vi "Car-tracking-poc.vi"() -> ()   [LabVIEW 2026]
uses:
  CTI-Grove/Examples/Sourcecode/cti-drivers-lv-visa-simple/Examples/Driver/Public/Digital Direction.ctl
  CTI-Grove/Examples/Sourcecode/cti-drivers-lv-visa-simple/Examples/Driver/CTIPicoVISA.lvlib
panel:
  out "RIGHT":bool
  out "CENTRE":bool
  out "LEFT":bool
  out "Identity":T1
  in  "stop":bool
  in  "VISA resource name in":refnum<visa-resource-name>="ASRL1::INSTR"
  out "error out":errorcluster
  # "https://wiki.seeedstudio.com/Grove-Passive-Buzzer/"
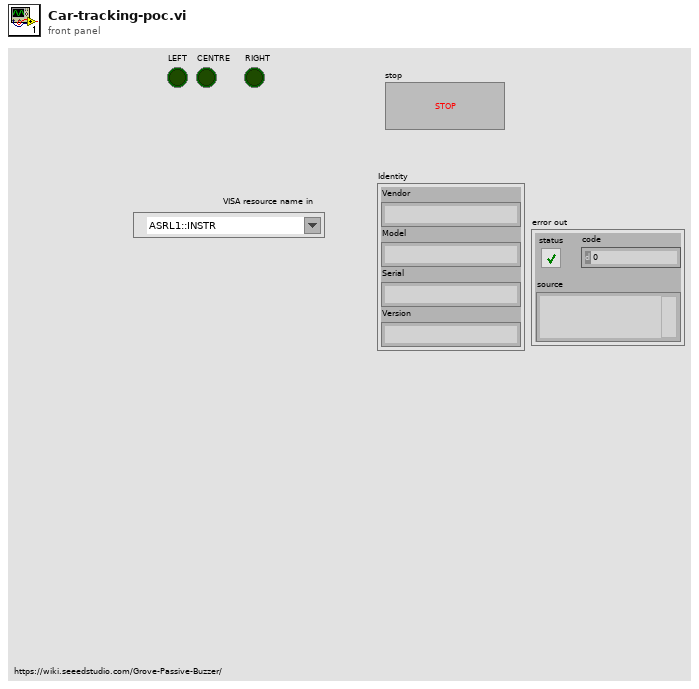
[diagram p1: front panel]
types:
  T1 = cluster{"Vendor":string, "Model":string, "Serial":string, "Version":string}
  T2 = typedef "CTIPicoVISA.lvlib/Digital Direction.ctl" = enum16{"In", "Out"}
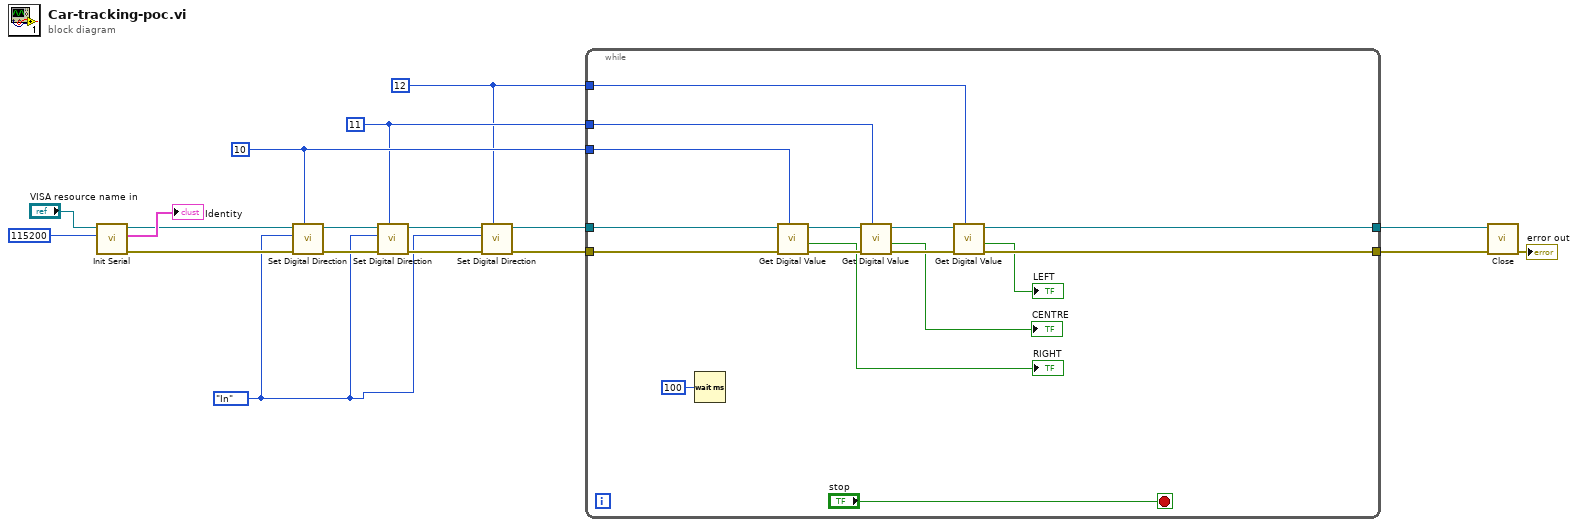
[diagram p0: block diagram]
diagram:
  w1 = 12 ("GPIO")
  w8 = 11 ("GPIO")
  w4 = Digital_Direction."In" ("Direction")
  w12 = 10 ("GPIO")
  n1 = call "Init Serial.vi"("Baud (115200)"=u32 115200, "VISA resource name in"="VISA resource name in") -> ("error out"=w13:errorcluster, "Identity"=→"Identity":T1, "VISA resource name Out"=w14:refnum<visa-resource-name>)  [unwired: 7 in]
  n2 = call "Set Digital Direction.vi"("GPIO"=w12, "error in (no error)"=w13, "Direction"=w4, "VISA resource name in"=w14) -> ("error out"=w10:errorcluster, "VISA resource name"=w11:refnum<visa-resource-name>)  [unwired: 6 in]
  n3 = call "Set Digital Direction.vi"("GPIO"=w8, "error in (no error)"=w10, "Direction"=w4, "VISA resource name in"=w11) -> ("error out"=w9:errorcluster, "VISA resource name"=w6:refnum<visa-resource-name>)  [unwired: 6 in]
  n4 = call "Set Digital Direction.vi"("GPIO"=w1, "error in (no error)"=w9, "Direction"=w4, "VISA resource name in"=w6) -> ("error out"=w7:errorcluster, "VISA resource name"=w5:refnum<visa-resource-name>)  [unwired: 6 in]
  n5 = while {
    tunnel: w12 -> [w22]
    tunnel: w5 -> [w32]
    tunnel: w7 -> [w28]
    tunnel: w8 -> [w23]
    tunnel: [w29] -> w3
    tunnel: [w25] -> w2
    tunnel: w1 -> [w24]
    stop <- "stop" stop-if-true
    n6 = Wait (ms)(milliseconds to wait=u32 100) -> ()  [unwired: 1 out]
    n7 = call "Get Digital Value.vi"("GPIO"=w22, "error in (no error)"=w28, "VISA resource name in"=w32) -> ("error out"=w27:errorcluster, "Value"=→"RIGHT":bool, "VISA resource name"=w31:refnum<visa-resource-name>)  [unwired: 6 in]
    n8 = call "Get Digital Value.vi"("GPIO"=w23, "error in (no error)"=w27, "VISA resource name in"=w31) -> ("error out"=w26:errorcluster, "Value"=→"CENTRE":bool, "VISA resource name"=w30:refnum<visa-resource-name>)  [unwired: 6 in]
    n9 = call "Get Digital Value.vi"("GPIO"=w24, "error in (no error)"=w26, "VISA resource name in"=w30) -> ("error out"=w25:errorcluster, "Value"=→"LEFT":bool, "VISA resource name"=w29:refnum<visa-resource-name>)  [unwired: 6 in]
  }
  n10 = call "Close.vi"("error in (no error)"=w2, "VISA resource name in"=w3) -> ("error out"=→"error out":errorcluster)  [unwired: 9 in]
